vi "create EIP channel.vi"(4 "subindex":i32, 6 "byte index":i32, 8 "Type":T2=enum."Consuming", 9 "Instance ID":u32, 10 "data type":T1, 11 "name":string) -> (3 "EthernetIP Channel out":refnum<class "EthernetIP Channel.lvclass">)   [LabVIEW 2013, in "EthernetIP Channel.lvclass"]
uses:
  EthernetIP Channel.lvclass
  configuration/assembly type.ctl
  <vilib>/NI/Tag Bus/tag/Data Type.ctl
  <vilib>/NI/Tag Bus/tag/tag descriptor.lvclass/tag descriptor.ctl
  <vilib>/NI/Tag Bus Module Framework/channel/TBM channel.lvclass/TBM channel.ctl
  EthernetIP Channel.lvclass/EthernetIP Channel.ctl
  <vilib>/NI/Tag Bus/tag/tag descriptor.lvclass
  <vilib>/NI/Tag Bus Module Framework/channel/TBM channel.lvclass
  configuration/EthernetIP configuration.lvclass
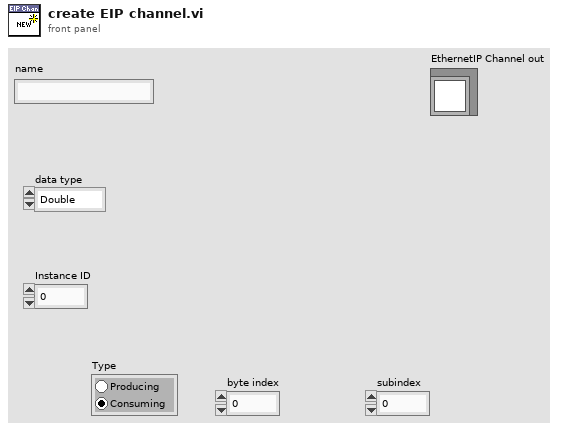
[diagram p1: front panel]
types:
  T1 = typedef "tag bus.lvlib/tag descriptor.lvclass/Data Type.ctl" = enum16{"Double", "Single", "I64", "I32", "I16", "I8", "U64", "U32", "U16", "U8", "Boolean", "String", "Array of Double", "Array of Single", "Array of I64", "Array of I32", "Array of I16", "Array of I8", "Array of U64", "Array of U32", "Array of U16", "Array of U8", "Array of Boolean", "Array of String"}
  T2 = typedef "EthernetIP configuration.lvclass/assembly type.ctl" = enum32{"Producing", "Consuming"}
  T3 = typedef "TBM channel.lvclass/channel classification.ctl" = enum16{"input data", "output data", "processing parameter", "processing result"}
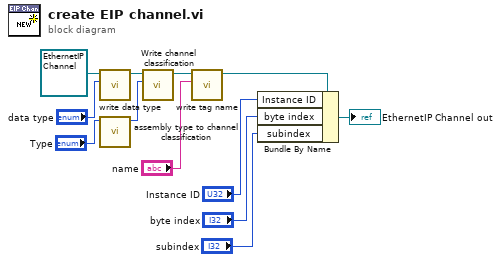
[diagram p0: block diagram]
diagram:
  n1 = call <vilib>:"write data type.vi"("data type"="data type", "system tag in"=refnum<class "EthernetIP Channel.lvclass"> refnum ("EthernetIP Channel in")) -> ("system tag out"=w10:refnum<class "EthernetIP Channel.lvclass">)  [unwired: 8 in, 1 out]
  n2 = call "assembly type to channel classification.vi"("Type"="Type") -> ("channel classification"=w4:T3)  [unwired: 10 in]
  n3 = call <vilib>:"Write channel classification.vi"("channel classification"=w4, "channel in"=w10) -> ("channel out"=w6:refnum<class "EthernetIP Channel.lvclass">)  [unwired: 8 in, 1 out]
  n4 = call <vilib>:"write tag name.vi"("name"="name", "system tag in"=w6) -> ("system tag out"=w11:refnum<class "EthernetIP Channel.lvclass">)  [unwired: 8 in, 1 out]
  n5 = Bundle By Name(cluster=w11, "Instance ID"="Instance ID", "byte index"="byte index", "subindex"="subindex") -> (→"EthernetIP Channel out":refnum<class "EthernetIP Channel.lvclass">)
